vi "GEA2 Serial Dryer Status.vi"(0 "Bytes Comm":u8[](array[numeric]), 5 "VISA resource name":refnum<visa-resource-name>, 7 "Dryer Status Serial Data In":T1) -> (8 "Dryer Status Serial Data Out":T1)   [LabVIEW 2014]
uses:
  Dryer Wilt/Type Definitions/WILT Dryer Com Port Info.ctl
  Dryer Wilt/Type Definitions/WILT Dryer Status Ctrl.ctl
  GEA2 Serial Globals Dryer.vi
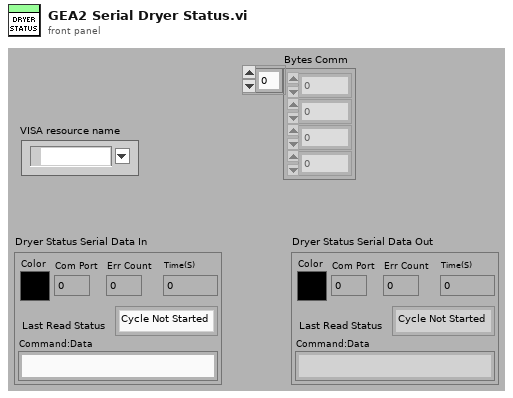
[diagram p1: front panel]
types:
  T1 = typedef "WILT Dryer Com Port Info.ctl" = cluster{"Color":u32, "Last Read Status":T2, "Command:Data":string, "Com Port":u8, "Time(S)":dbl, "Err Count":u32}
  T2 = typedef "WILT Dryer Status Ctrl.ctl" = enum16{"Cycle Not Started", "Cycle Running", "Paused", "Cycle Completed", "Eval Mode Entered", "Err", "Pause (No GEA2)"}
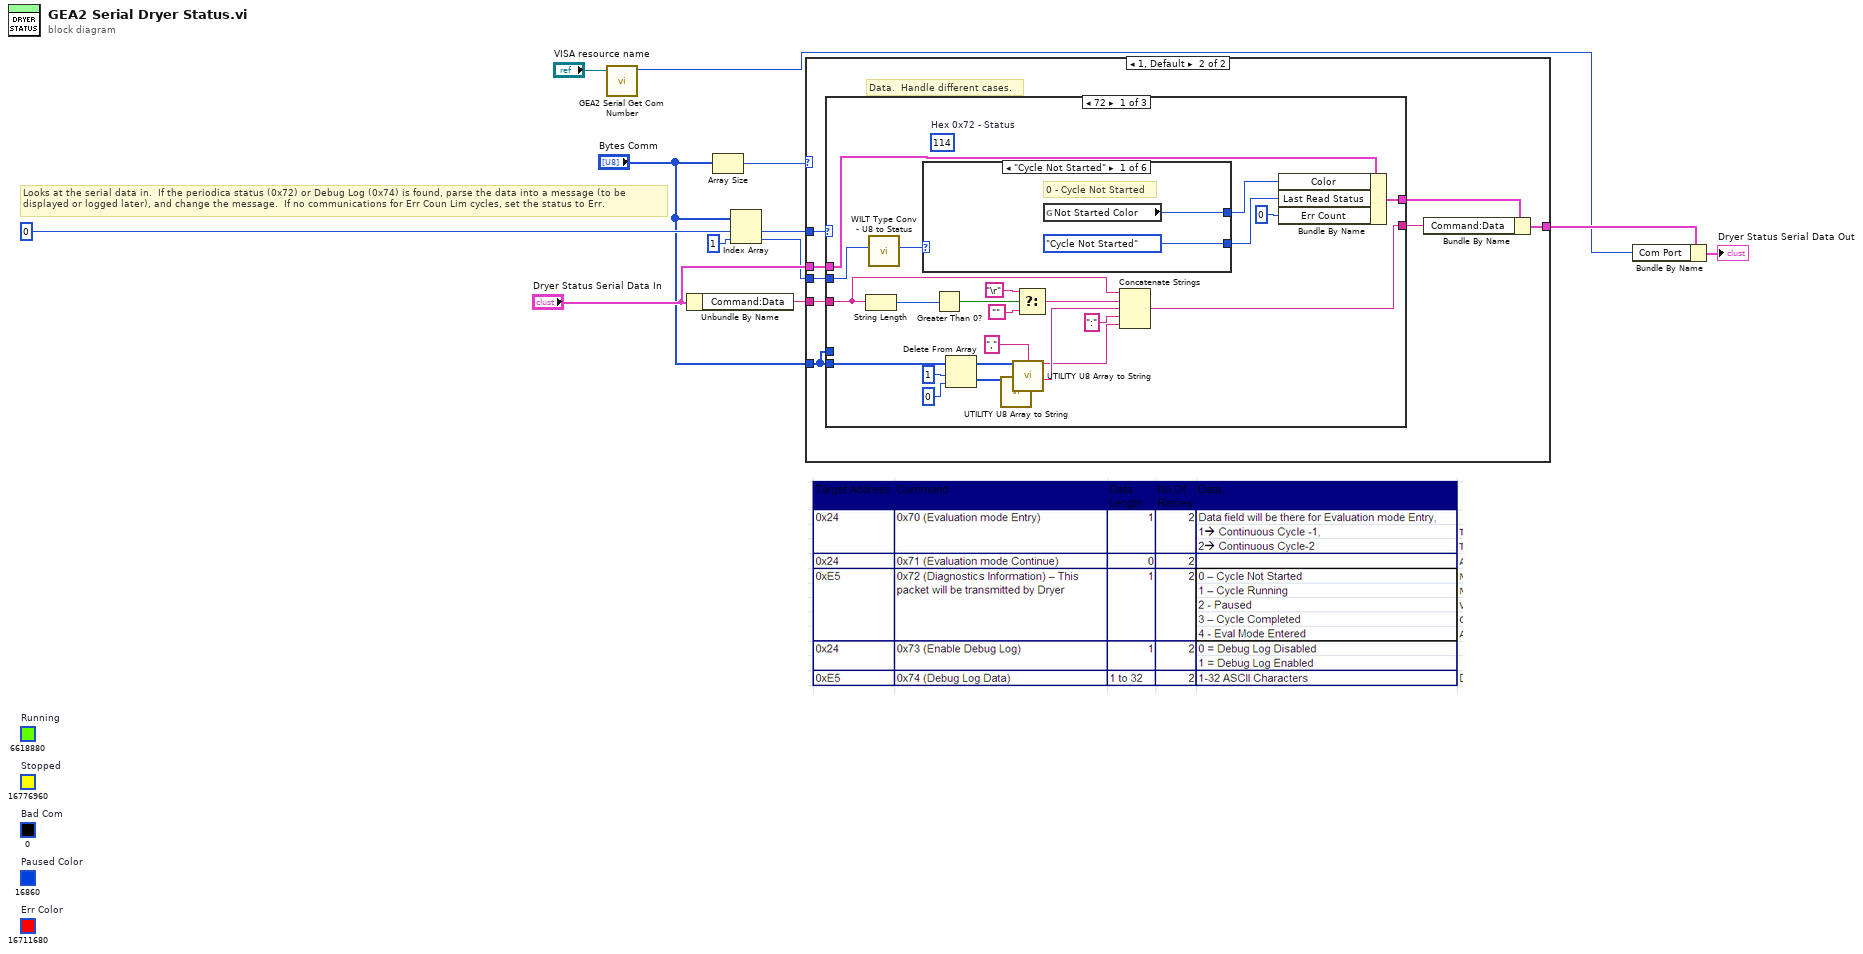
[diagram p0: block diagram]
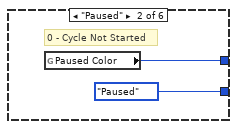
[diagram p3: hidden frame]
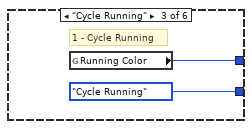
[diagram p4: hidden frame]
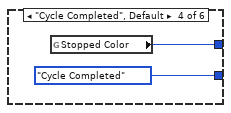
[diagram p5: hidden frame]
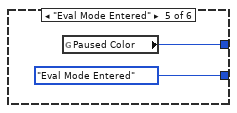
[diagram p6: hidden frame]
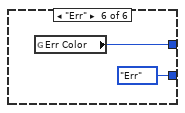
[diagram p7: hidden frame]
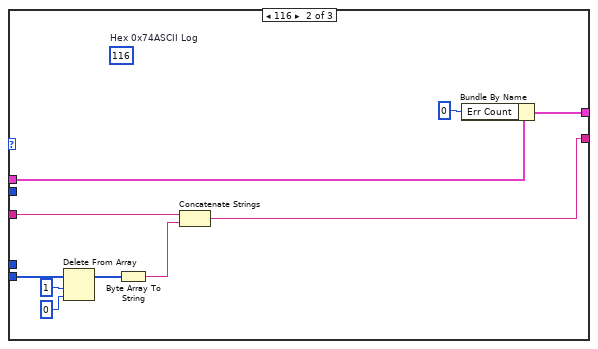
[diagram p8: hidden frame]
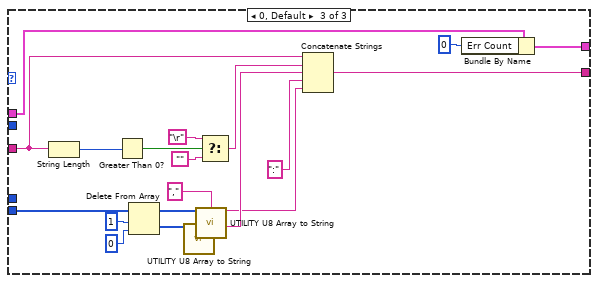
[diagram p9: hidden frame]
diagram:
  (unwired) u32 16711680  # Err Color
  (unwired) u32 16860  # Paused Color
  (unwired) u32 0  # Bad Com
  (unwired) u32 6618880  # Running
  (unwired) u32 16776960  # Stopped
  # "Looks at the serial data in.  If the periodica status (0x72) or Debug Log (0x74) is found, parse the data into a message (to be \ndisplayed or logged later), and change the message.  If no communications for Err Coun Lim cycles, set the status to Err."
  n1 = call "GEA2 Serial Get Com Number.vi"("ComPort Local Copy"="VISA resource name") -> ("Com Num"=w1:u8)  [unwired: 10 in]
  n2 = Unbundle By Name("Dryer Status Serial Data In") -> ("Command:Data"=w3:string)
  n3 = Array Size(array="Bytes Comm") -> (size(s)=w9:i32)
  n4 = Index Array(array="Bytes Comm", index #1=0 ("index"), index #2=1 ("index")) -> (element #1=w6:u8, element #2=w7:u8)
  n5 = case shown="1, Default" w9 {
    tunnel: w7 -> [_ w18]
    tunnel: w6 -> [_ w17]
    tunnel: "Dryer Status Serial Data In" -> [w13 w21]
    tunnel: [w13 w19] -> w5
    tunnel: "Bytes Comm" -> [_ w15]
    tunnel: w3 -> [_ w16]
    frame 0 {
      # "No data."
    }
    frame 1, Default {
      # "Data.  Handle different cases."
      n6 = case shown="72" w17 {
        tunnel: w18 -> [w23 _ _]
        tunnel: w21 -> [w44 w59 w68]
        tunnel: [w43 w58 w67] -> w20
        tunnel: w15 -> [_ _ _]
        tunnel: w16 -> [w27 w62 w72]
        tunnel: w15 -> [w28 w63 w73]
        tunnel: [w25 w60 w70] -> w14
        frame 114 {
          (unwired) 114  # Hex 0x72 - Status
          n7 = String Length(string=w27) -> (length=w35:i32)
          n8 = call "WILT Type Conv - U8 to Status.vi"("Byte Val"=w23) -> ("Status"=w24:T2)  [unwired: 10 in]
          n9 = case shown="\"Cycle Not Started\"" w24 {
            tunnel: [w45 w48 w50 w51 w54 w56] -> w41
            tunnel: [WILT_Dryer_Status_Ctrl."Cycle Not Started" ("Status") WILT_Dryer_Status_Ctrl."Paused" ("Status") WILT_Dryer_Status_Ctrl."Cycle Running" ("Status") WILT_Dryer_Status_Ctrl."Cycle Completed" ("Status") WILT_Dryer_Status_Ctrl."Eval Mode Entered" ("Status") WILT_Dryer_Status_Ctrl."Err" ("Status")] -> w42
            frame "Cycle Not Started" {
              # "0 - Cycle Not Started"
              n10 = global read "GEA2 Serial Globals Dryer.vi" "Not Started Color"() -> (w45:u32)
            }
            frame "Paused" {
              # "0 - Cycle Not Started"
              n11 = global read "GEA2 Serial Globals Dryer.vi" "Paused Color"() -> (w48:u32)
            }
            frame "Cycle Running" {
              # "1 - Cycle Running"
              n12 = global read "GEA2 Serial Globals Dryer.vi" "Running Color"() -> (w50:u32)
            }
            frame "Cycle Completed", Default {
              n13 = global read "GEA2 Serial Globals Dryer.vi" "Stopped Color"() -> (w51:u32)
            }
            frame "Eval Mode Entered" {
              n14 = global read "GEA2 Serial Globals Dryer.vi" "Paused Color"() -> (w54:u32)
            }
            frame "Err" {
              n15 = global read "GEA2 Serial Globals Dryer.vi" "Err Color"() -> (w56:u32)
            }
          }
          n16 = Greater Than 0?(x=w35) -> (x > 0?=w36:bool)
          n17 = Delete From Array(array=w28, length=1, index=0) -> (deleted portion=w29:u8[], array with subset deleted=w26:u8[])
          n18 = call "UTILITY U8 Array to String.vi"("U8 Data"=w29) -> ("String"=w32:string)  [unwired: 14 in]
          n19 = call "UTILITY U8 Array to String.vi"("U8 Data"=w26, "Delimiter(_)"=",") -> ("String"=w30:string)  [unwired: 13 in]
          n20 = Select(t="\r", s=w36, f="") -> (s? t:f=w39:string)
          n21 = Concatenate Strings(w27, w39, w32, ":" ("string"), w30) -> (w25:string)
          n22 = Bundle By Name(cluster=w44, "Color"=w41, "Last Read Status"=w42, "Err Count"=u32 0) -> (w43:T1)
        }
        frame 116 {
          (unwired) 116  # Hex 0x74ASCII Log
          n23 = Delete From Array(array=w63, length=1, index=0) -> (array with subset deleted=w61:u8[])  [unwired: 1 out]
          n24 = Byte Array To String(unsigned byte array=w61) -> (string=w64:string)
          n25 = Concatenate Strings(w62, w64) -> (w60:string)
          n26 = Bundle By Name(cluster=w59, "Err Count"=u32 0) -> (w58:T1)
        }
        frame 0, Default {
          n27 = String Length(string=w72) -> (length=w80:i32)
          n28 = Greater Than 0?(x=w80) -> (x > 0?=w81:bool)
          n29 = Delete From Array(array=w73, length=1, index=0) -> (deleted portion=w74:u8[], array with subset deleted=w71:u8[])
          n30 = call "UTILITY U8 Array to String.vi"("U8 Data"=w74) -> ("String"=w77:string)  [unwired: 14 in]
          n31 = call "UTILITY U8 Array to String.vi"("U8 Data"=w71, "Delimiter(_)"=",") -> ("String"=w75:string)  [unwired: 13 in]
          n32 = Select(t="\r", s=w81, f="") -> (s? t:f=w84:string)
          n33 = Concatenate Strings(w72, w84, w77, ":" ("string"), w75) -> (w70:string)
          n34 = Bundle By Name(cluster=w68, "Err Count"=u32 0) -> (w67:T1)
        }
      }
      n35 = Bundle By Name(cluster=w20, "Command:Data"=w14) -> (w19:T1)
    }
  }
  n36 = Bundle By Name(cluster=w5, "Com Port"=w1) -> (→"Dryer Status Serial Data Out":T1)
